vi "Defragment TDMS.vi"() -> ()   [LabVIEW 2016]
panel:
  in  "File Path Control":path
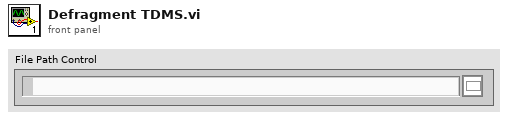
[diagram p1: front panel]
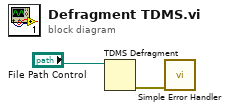
[diagram p0: block diagram]
diagram:
  n1 = TDMS Defragment(7:"File Path Control") -> (0:w1:errorcluster)  [unwired: 1 in]
  n2 = call <vilib>:"Simple Error Handler.vi"("error in (no error)"=w1) -> ()  [unwired: 4 in, 5 out]
